vi "AttackedSquares.vi"(10 "Turn":T2, 11 "Input Squares":T1[][](array[typedef])) -> (3 "Attacked Squares":bool[][](array[boolean]))   [LabVIEW 2019]
doc: "This VI creates virtual chessboard with squares attacked by player that made last move"
uses:
  #typedef_Color.ctl
  #typedef_SquareType.ctl
  #typedef_Piece.ctl
  #typedef_PieceType.ctl
panel:
  out "?":u16[][](array[ring])
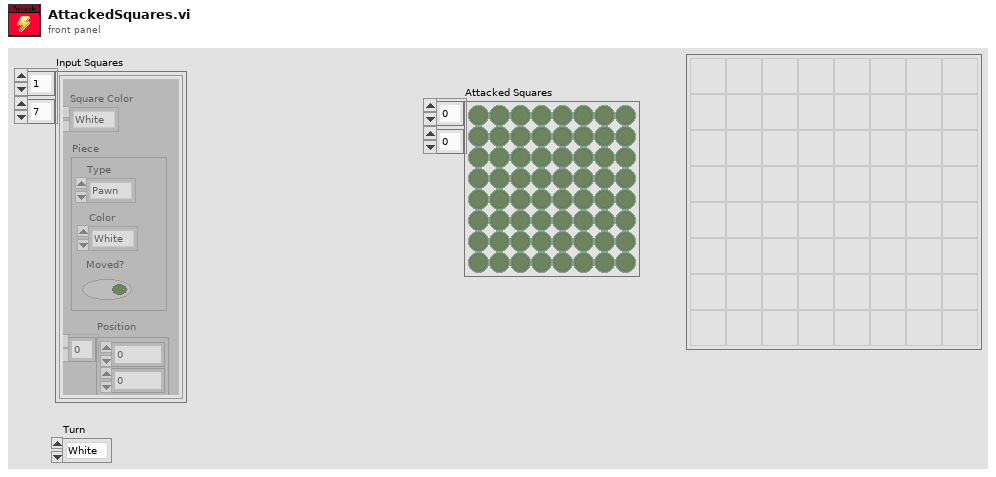
[diagram p1: front panel]
types:
  T1 = typedef "#typedef_SquareType.ctl" = cluster{"Square Color":T2, "Position":i32[], "Piece":T3}
  T2 = typedef "#typedef_Color.ctl" = enum16{"White", "Black"}
  T3 = typedef "#typedef_Piece.ctl" = cluster{"Type":T4, "Color":T2, "Moved?":bool}
  T4 = typedef "#typedef_PieceType.ctl" = enum16{"None", "Pawn", "Knight", "Bishop", "Rook", "Queen", "King"}
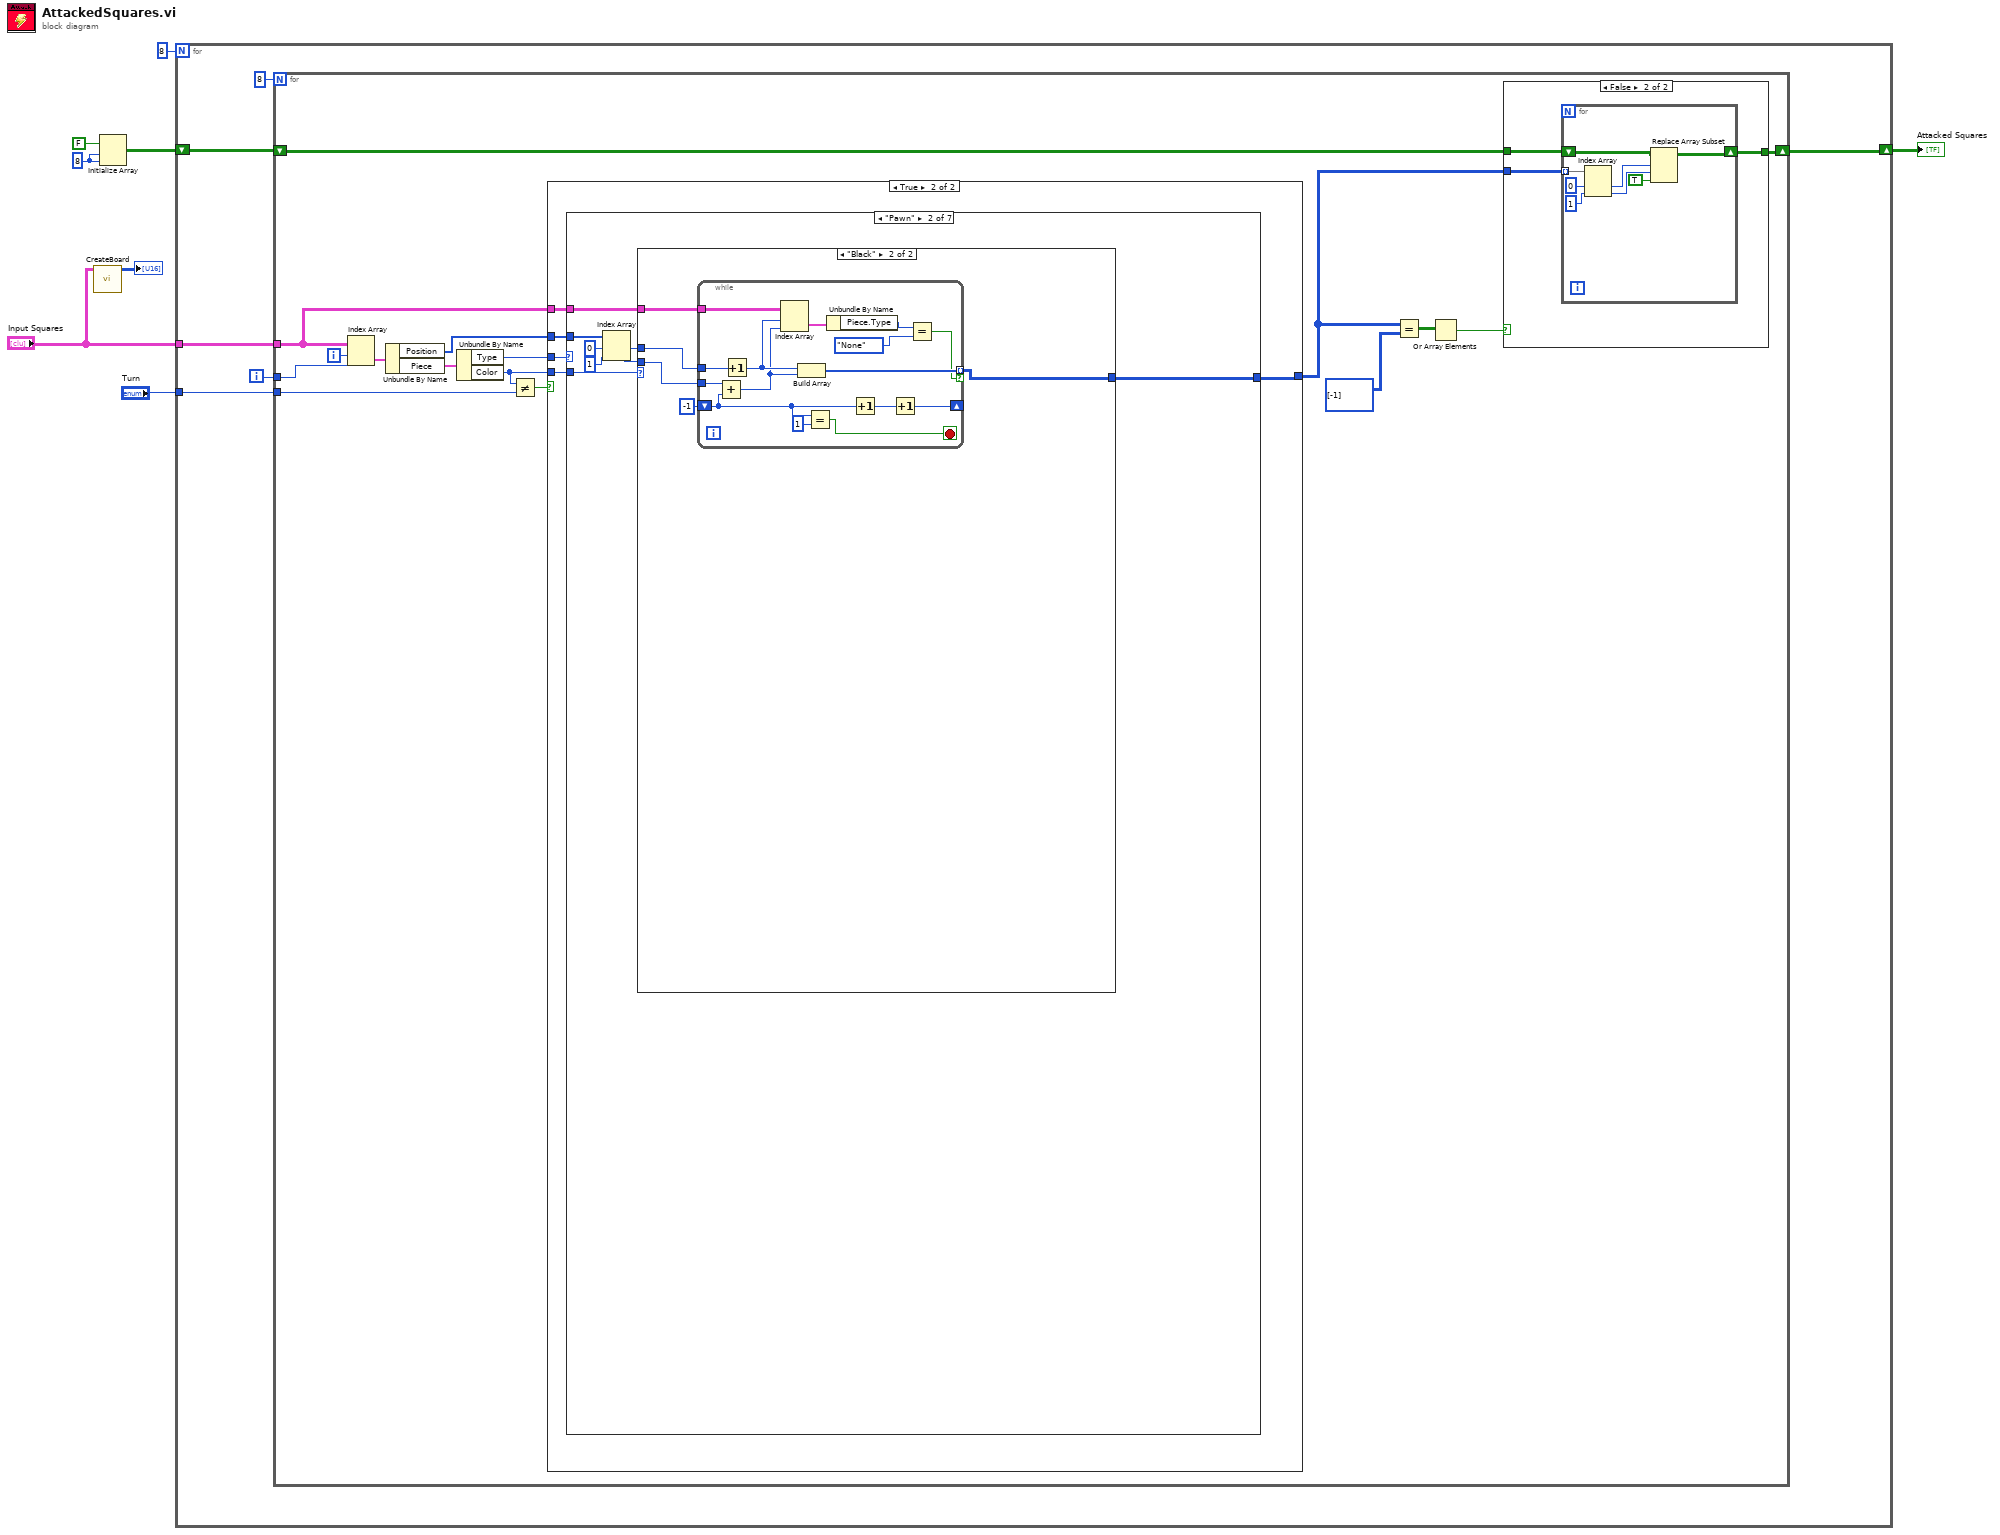
[diagram p0: block diagram]
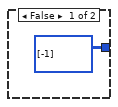
[diagram p3: hidden frame]
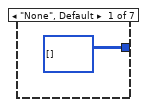
[diagram p4: hidden frame]
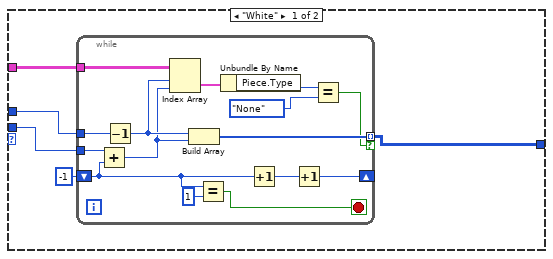
[diagram p5: hidden frame]
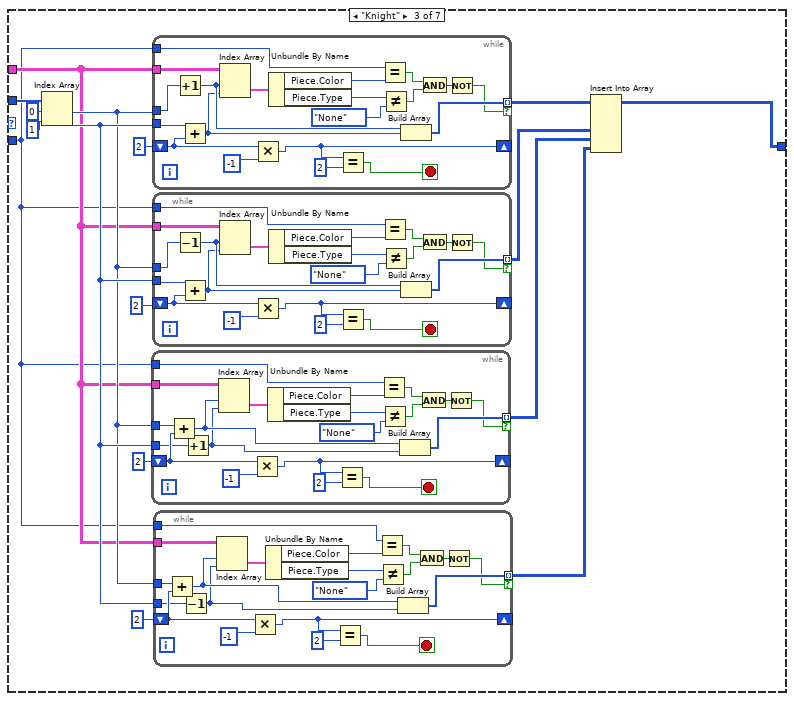
[diagram p6: hidden frame]
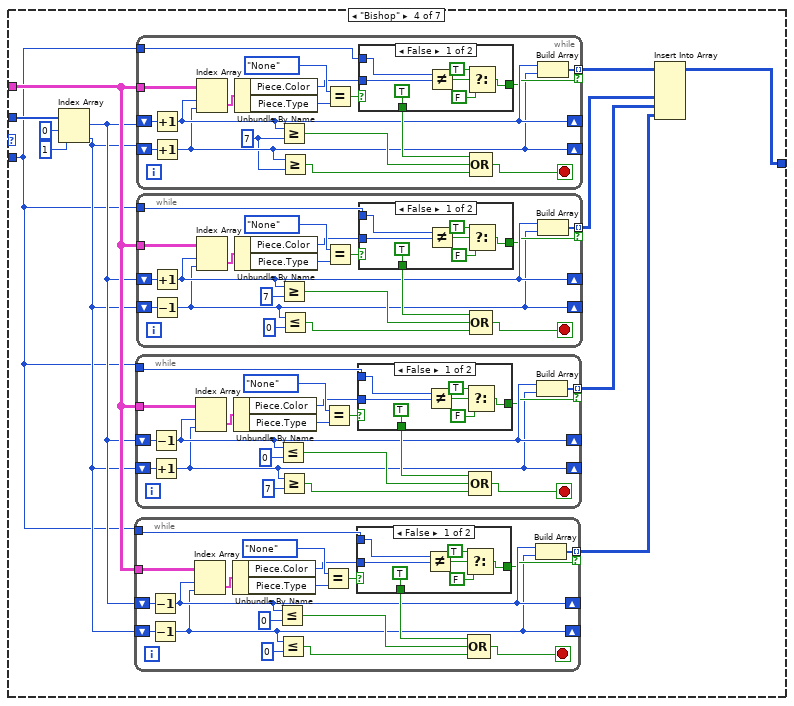
[diagram p7: hidden frame]
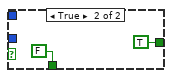
[diagram p8: hidden frame]
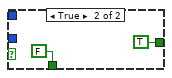
[diagram p9: hidden frame]
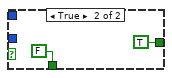
[diagram p10: hidden frame]
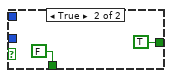
[diagram p11: hidden frame]
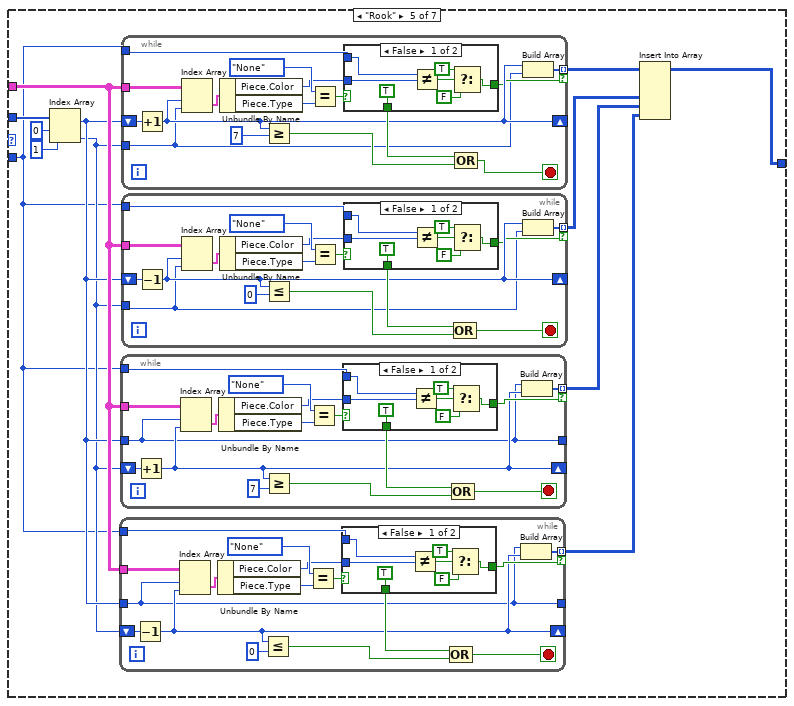
[diagram p12: hidden frame]
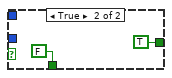
[diagram p13: hidden frame]
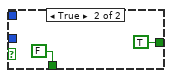
[diagram p14: hidden frame]
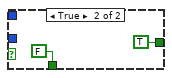
[diagram p15: hidden frame]
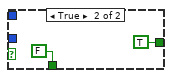
[diagram p16: hidden frame]
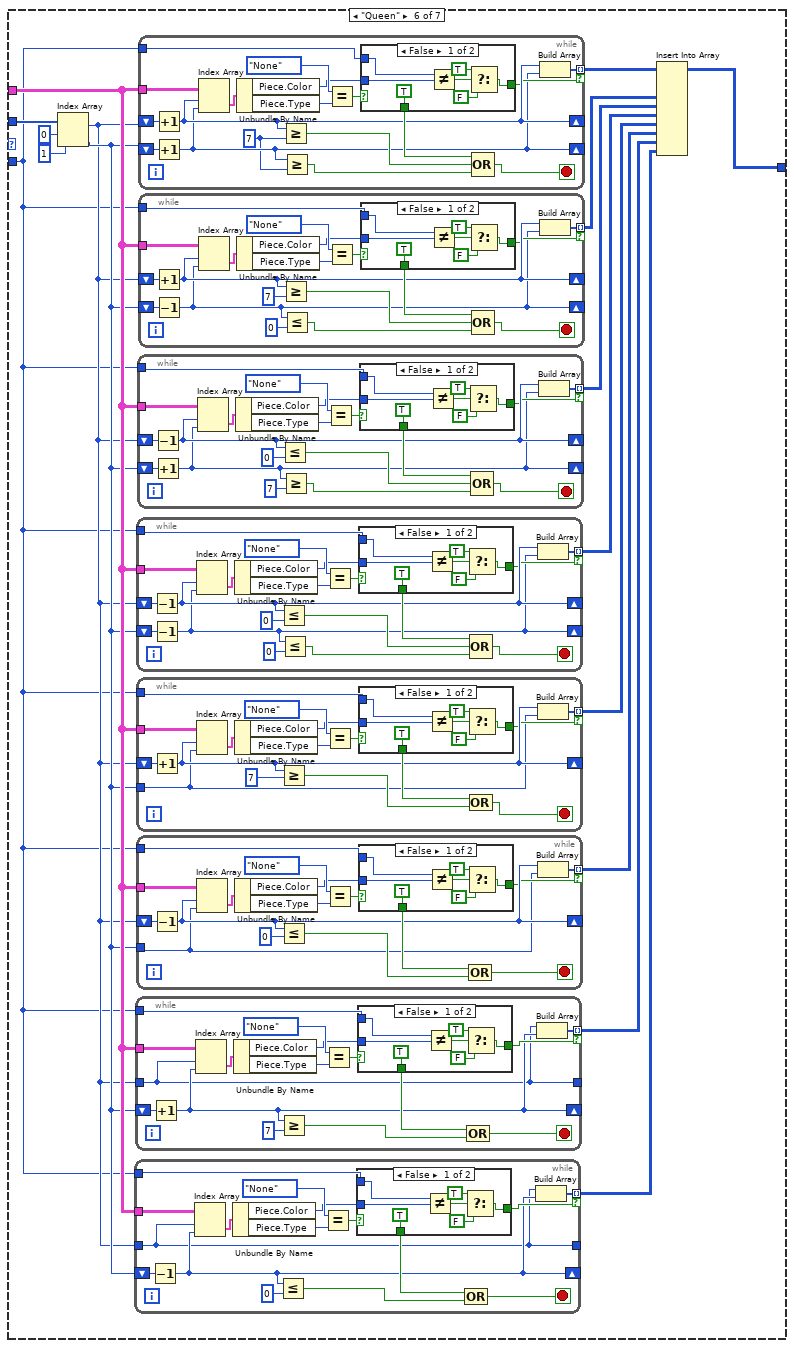
[diagram p17: hidden frame]
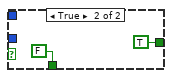
[diagram p18: hidden frame]
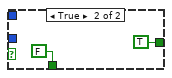
[diagram p19: hidden frame]
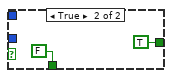
[diagram p20: hidden frame]
diagram:
  w5 = 8 ("dimension size")
  n1 = call "CreateBoard.vi"("Squares type"="Input Squares") -> ("Board"=→"?":u16[][])  [unwired: 10 in]
  n2 = Initialize Array(FALSE, w5, w5) -> (w6:bool[][])
  n3 = for {
    N: 8 -> [_]
    tunnel: "Input Squares" -> [w14]
    tunnel: "Turn" -> [w13]
    shift-right: [w10] -> w7
    shift-left: w6 -> [w11]
    i -> [w12]
    n4 = for {
      N: 8 -> [_]
      tunnel: w14 -> [w30]
      tunnel: w13 -> [w25]
      tunnel: w12 -> [w21]
      shift-right: [w15] -> w10
      shift-left: w11 -> [w17]
      i -> [w22]
      n5 = Index Array(array=w30, index (row)=w22, index (col)=w21) -> (element=w23:T1)
      n6 = Unbundle By Name(w23) -> ("Position"=w28:i32[], "Piece"=w24:T3)
      n7 = Unbundle By Name(w24) -> ("Type"=w27:T4, "Color"=w29:T2)
      n8 = Not Equal?(x=w29, y=w25) -> (x != y?=w26:bool)
      n9 = case shown="True" w26 {
        tunnel: w27 -> [_ w48]
        tunnel: w28 -> [_ w47]
        tunnel: w29 -> [_ w46]
        tunnel: w30 -> [_ w45]
        tunnel: [i32[][] [[-1]] w44] -> w16
        frame False {
        }
        frame True {
          n10 = case shown="\"Pawn\"" w48 {
            tunnel: w47 -> [_ w54 w100 w203 w326 w442 w669]
            tunnel: w46 -> [_ w57 w99 w195 w318 w434 w661]
            tunnel: w45 -> [_ w51 w101 w198 w321 w437 w664]
            tunnel: [i32[][] [] w50 w98 w194 w317 w429 w656] -> w44
            frame "None", Default {
            }
            frame "Pawn" {
              n11 = Index Array(array=w54, index #1=0 ("index"), index #2=1 ("index")) -> (element #1=w53:i32, element #2=w52:i32)
              n12 = case shown="\"Black\"" w57 {
                tunnel: w53 -> [w61 w81]
                tunnel: w52 -> [w60 w80]
                tunnel: w51 -> [w59 w79]
                tunnel: [w58 w78] -> w50
                frame "White" {
                  n13 = while {
                    tunnel: w61 -> [w73]
                    tunnel: w60 -> [w72]
                    tunnel: w59 -> [w70]
                    tunnel: [w64] -> w58 mode=indexing if=w63
                    shift-right: [w76] -> _
                    shift-left: -1 ("index") -> [w71]
                    stop <- w74 stop-if-true
                    n14 = Add(x=w72, y=w71) -> (x+y=w65:i32)
                    n15 = Decrement(x=w73) -> (x-1=w66:i32)
                    n16 = Index Array(array=w70, index (row)=w66, index (col)=w65) -> (element=w69:T1)
                    n17 = Build Array(w66, w65) -> (w64:i32[])
                    n18 = Equal?(x=w71, y=1) -> (x = y?=w74:bool)
                    n19 = Unbundle By Name(w69) -> ("Piece.Type"=w68:T4)
                    n20 = Increment(x=w71) -> (x+1=w77:i32)
                    n21 = Increment(x=w77) -> (x+1=w76:i32)
                    n22 = Equal?(x=w68, y=#typedef_PieceType."None") -> (x = y?=w63:bool)
                  }
                }
                frame "Black" {
                  n23 = while {
                    tunnel: w81 -> [w93]
                    tunnel: w80 -> [w92]
                    tunnel: w79 -> [w90]
                    tunnel: [w84] -> w78 mode=indexing if=w83
                    shift-right: [w96] -> _
                    shift-left: -1 ("index") -> [w91]
                    stop <- w94 stop-if-true
                    n24 = Add(x=w92, y=w91) -> (x+y=w85:i32)
                    n25 = Increment(x=w93) -> (x+1=w86:i32)
                    n26 = Index Array(array=w90, index (row)=w86, index (col)=w85) -> (element=w89:T1)
                    n27 = Build Array(w86, w85) -> (w84:i32[])
                    n28 = Equal?(x=w91, y=1) -> (x = y?=w94:bool)
                    n29 = Unbundle By Name(w89) -> ("Piece.Type"=w88:T4)
                    n30 = Increment(x=w91) -> (x+1=w97:i32)
                    n31 = Increment(x=w97) -> (x+1=w96:i32)
                    n32 = Equal?(x=w88, y=#typedef_PieceType."None") -> (x = y?=w83:bool)
                  }
                }
              }
            }
            frame "Knight" {
              n33 = Index Array(array=w100, index #1=0 ("index"), index #2=1 ("index")) -> (element #1=w106:i32, element #2=w107:i32)
              n34 = while {
                tunnel: w101 -> [w153]
                tunnel: w106 -> [w140]
                tunnel: w107 -> [w138]
                shift-right: [w146] -> _
                shift-left: 2 -> [w139]
                tunnel: [w143] -> w103 mode=indexing if=w141
                tunnel: w99 -> [w134]
                stop <- w144 stop-if-true
                n35 = Add(x=w140, y=w139) -> (x+y=w137:i32)
                n36 = Increment(x=w138) -> (x+1=w136:i32)
                n37 = Index Array(array=w153, index (row)=w137, index (col)=w136) -> (element=w151:T1)
                n38 = Multiply(x=w139, y=-1) -> (x*y=w146:i32)
                n39 = Unbundle By Name(w151) -> ("Piece.Color"=w150:T2, "Piece.Type"=w149:T4)
                n40 = Equal?(x=w146, y=2) -> (x = y?=w144:bool)
                n41 = Equal?(x=w134, y=w150) -> (x = y?=w148:bool)
                n42 = Not Equal?(x=w149, y=#typedef_PieceType."None") -> (x != y?=w147:bool)
                n43 = Build Array(w137, w136) -> (w143:i32[])
                n44 = And(x=w148, y=w147) -> (x .and. y?=w142:bool)
                n45 = Not(x=w142) -> (.not. x?=w141:bool)
              }
              n46 = while {
                tunnel: w101 -> [w193]
                tunnel: w106 -> [w189]
                tunnel: w107 -> [w190]
                shift-right: [w183] -> _
                shift-left: 2 -> [w191]
                tunnel: [w178] -> w105 mode=indexing if=w176
                tunnel: w99 -> [w174]
                stop <- w181 stop-if-true
                n47 = Increment(x=w189) -> (x+1=w180:i32)
                n48 = Add(x=w190, y=w191) -> (x+y=w179:i32)
                n49 = Index Array(array=w193, index (row)=w180, index (col)=w179) -> (element=w188:T1)
                n50 = Multiply(x=w191, y=-1) -> (x*y=w183:i32)
                n51 = Unbundle By Name(w188) -> ("Piece.Color"=w187:T2, "Piece.Type"=w186:T4)
                n52 = Equal?(x=w183, y=2) -> (x = y?=w181:bool)
                n53 = Equal?(x=w174, y=w187) -> (x = y?=w185:bool)
                n54 = Not Equal?(x=w186, y=#typedef_PieceType."None") -> (x != y?=w184:bool)
                n55 = Build Array(w180, w179) -> (w178:i32[])
                n56 = And(x=w185, y=w184) -> (x .and. y?=w177:bool)
                n57 = Not(x=w177) -> (.not. x?=w176:bool)
              }
              n58 = while {
                tunnel: w101 -> [w173]
                tunnel: w106 -> [w169]
                tunnel: w107 -> [w170]
                shift-right: [w163] -> _
                shift-left: 2 -> [w171]
                tunnel: [w158] -> w104 mode=indexing if=w156
                tunnel: w99 -> [w154]
                stop <- w161 stop-if-true
                n59 = Decrement(x=w169) -> (x-1=w160:i32)
                n60 = Add(x=w170, y=w171) -> (x+y=w159:i32)
                n61 = Index Array(array=w173, index (row)=w160, index (col)=w159) -> (element=w168:T1)
                n62 = Multiply(x=w171, y=-1) -> (x*y=w163:i32)
                n63 = Unbundle By Name(w168) -> ("Piece.Color"=w167:T2, "Piece.Type"=w166:T4)
                n64 = Equal?(x=w163, y=2) -> (x = y?=w161:bool)
                n65 = Equal?(x=w154, y=w167) -> (x = y?=w165:bool)
                n66 = Not Equal?(x=w166, y=#typedef_PieceType."None") -> (x != y?=w164:bool)
                n67 = Build Array(w160, w159) -> (w158:i32[])
                n68 = And(x=w165, y=w164) -> (x .and. y?=w157:bool)
                n69 = Not(x=w157) -> (.not. x?=w156:bool)
              }
              n70 = while {
                tunnel: w101 -> [w133]
                tunnel: w106 -> [w120]
                tunnel: w107 -> [w118]
                shift-right: [w126] -> _
                shift-left: 2 -> [w119]
                tunnel: [w123] -> w102 mode=indexing if=w121
                tunnel: w99 -> [w114]
                stop <- w124 stop-if-true
                n71 = Add(x=w120, y=w119) -> (x+y=w117:i32)
                n72 = Decrement(x=w118) -> (x-1=w116:i32)
                n73 = Index Array(array=w133, index (row)=w117, index (col)=w116) -> (element=w131:T1)
                n74 = Multiply(x=w119, y=-1) -> (x*y=w126:i32)
                n75 = Unbundle By Name(w131) -> ("Piece.Color"=w130:T2, "Piece.Type"=w129:T4)
                n76 = Equal?(x=w126, y=2) -> (x = y?=w124:bool)
                n77 = Equal?(x=w114, y=w130) -> (x = y?=w128:bool)
                n78 = Not Equal?(x=w129, y=#typedef_PieceType."None") -> (x != y?=w127:bool)
                n79 = Build Array(w117, w116) -> (w123:i32[])
                n80 = And(x=w128, y=w127) -> (x .and. y?=w122:bool)
                n81 = Not(x=w122) -> (.not. x?=w121:bool)
              }
              n82 = Insert Into Array(array=w105, new element #1=w104, new element #2=w103, new element #3=w102) -> (w98:i32[][])  [unwired: 2 in]
            }
            frame "Bishop" {
              n83 = Index Array(array=w203, index #1=0 ("index (row)"), index #2=1 ("index")) -> (element #1=w197:i32, element #2=w196:i32)
              n84 = while {
                tunnel: w198 -> [w222]
                shift-right: [w211] -> _
                shift-left: w197 -> [w223]
                shift-right: [w208] -> _
                shift-left: w196 -> [w224]
                tunnel: [w210] -> w199 mode=indexing if=w209
                tunnel: w195 -> [w206]
                stop <- w212 stop-if-true
                n85 = Decrement(x=w223) -> (x-1=w211:i32)
                n86 = Decrement(x=w224) -> (x-1=w208:i32)
                n87 = Index Array(array=w222, index (row)=w211, index (col)=w208) -> (element=w221:T1)
                n88 = Unbundle By Name(w221) -> ("Piece.Color"=w217:T2, "Piece.Type"=w220:T4)
                n89 = Less Or Equal?(x=w211, y=0) -> (x <= y?=w214:bool)
                n90 = Less Or Equal?(x=w208, y=0) -> (x <= y?=w213:bool)
                n91 = Equal?(x=#typedef_PieceType."None", y=w220) -> (x = y?=w218:bool)
                n92 = case shown="False" w218 {
                  tunnel: w217 -> [w231 _]
                  tunnel: [TRUE FALSE] -> w215
                  tunnel: [w226 TRUE] -> w209
                  tunnel: w206 -> [w225 _]
                  frame False {
                    n93 = Not Equal?(x=w225, y=w231) -> (x != y?=w229:bool)
                    n94 = Select(t=TRUE, s=w229, f=FALSE) -> (s? t:f=w226:bool)
                  }
                  frame True {
                  }
                }
                n95 = Compound Arithmetic op=OR(w215, w214, w213) -> (w212:bool)
                n96 = Build Array(w211, w208) -> (w210:i32[])
              }
              n97 = while {
                tunnel: w198 -> [w250]
                shift-right: [w239] -> _
                shift-left: w197 -> [w251]
                shift-right: [w236] -> _
                shift-left: w196 -> [w252]
                tunnel: [w238] -> w200 mode=indexing if=w237
                tunnel: w195 -> [w234]
                stop <- w240 stop-if-true
                n98 = Decrement(x=w251) -> (x-1=w239:i32)
                n99 = Increment(x=w252) -> (x+1=w236:i32)
                n100 = Index Array(array=w250, index (row)=w239, index (col)=w236) -> (element=w249:T1)
                n101 = Unbundle By Name(w249) -> ("Piece.Color"=w245:T2, "Piece.Type"=w248:T4)
                n102 = Less Or Equal?(x=w239, y=0) -> (x <= y?=w242:bool)
                n103 = Greater Or Equal?(x=w236, y=7) -> (x >= y?=w241:bool)
                n104 = Equal?(x=#typedef_PieceType."None", y=w248) -> (x = y?=w246:bool)
                n105 = case shown="False" w246 {
                  tunnel: w245 -> [w259 _]
                  tunnel: [TRUE FALSE] -> w243
                  tunnel: [w254 TRUE] -> w237
                  tunnel: w234 -> [w253 _]
                  frame False {
                    n106 = Not Equal?(x=w253, y=w259) -> (x != y?=w257:bool)
                    n107 = Select(t=TRUE, s=w257, f=FALSE) -> (s? t:f=w254:bool)
                  }
                  frame True {
                  }
                }
                n108 = Compound Arithmetic op=OR(w243, w242, w241) -> (w240:bool)
                n109 = Build Array(w239, w236) -> (w238:i32[])
              }
              n110 = while {
                tunnel: w198 -> [w305]
                shift-right: [w295] -> _
                shift-left: w197 -> [w306]
                shift-right: [w292] -> _
                shift-left: w196 -> [w307]
                tunnel: [w294] -> w202 mode=indexing if=w293
                tunnel: w195 -> [w290]
                stop <- w296 stop-if-true
                w291 = 7 ("y")
                n111 = Increment(x=w306) -> (x+1=w295:i32)
                n112 = Increment(x=w307) -> (x+1=w292:i32)
                n113 = Index Array(array=w305, index (row)=w295, index (col)=w292) -> (element=w304:T1)
                n114 = Unbundle By Name(w304) -> ("Piece.Color"=w300:T2, "Piece.Type"=w303:T4)
                n115 = Greater Or Equal?(x=w295, y=w291) -> (x >= y?=w298:bool)
                n116 = Greater Or Equal?(x=w292, y=w291) -> (x >= y?=w297:bool)
                n117 = Equal?(x=#typedef_PieceType."None", y=w303) -> (x = y?=w301:bool)
                n118 = case shown="False" w301 {
                  tunnel: w300 -> [w314 _]
                  tunnel: [TRUE FALSE] -> w299
                  tunnel: [w309 TRUE] -> w293
                  tunnel: w290 -> [w308 _]
                  frame False {
                    n119 = Not Equal?(x=w308, y=w314) -> (x != y?=w312:bool)
                    n120 = Select(t=TRUE, s=w312, f=FALSE) -> (s? t:f=w309:bool)
                  }
                  frame True {
                  }
                }
                n121 = Compound Arithmetic op=OR(w299, w298, w297) -> (w296:bool)
                n122 = Build Array(w295, w292) -> (w294:i32[])
              }
              n123 = while {
                tunnel: w198 -> [w278]
                shift-right: [w267] -> _
                shift-left: w197 -> [w279]
                shift-right: [w264] -> _
                shift-left: w196 -> [w280]
                tunnel: [w266] -> w201 mode=indexing if=w265
                tunnel: w195 -> [w262]
                stop <- w268 stop-if-true
                n124 = Increment(x=w279) -> (x+1=w267:i32)
                n125 = Decrement(x=w280) -> (x-1=w264:i32)
                n126 = Index Array(array=w278, index (row)=w267, index (col)=w264) -> (element=w277:T1)
                n127 = Unbundle By Name(w277) -> ("Piece.Color"=w273:T2, "Piece.Type"=w276:T4)
                n128 = Greater Or Equal?(x=w267, y=7) -> (x >= y?=w270:bool)
                n129 = Less Or Equal?(x=w264, y=0) -> (x <= y?=w269:bool)
                n130 = Equal?(x=#typedef_PieceType."None", y=w276) -> (x = y?=w274:bool)
                n131 = case shown="False" w274 {
                  tunnel: w273 -> [w287 _]
                  tunnel: [TRUE FALSE] -> w271
                  tunnel: [w282 TRUE] -> w265
                  tunnel: w262 -> [w281 _]
                  frame False {
                    n132 = Not Equal?(x=w281, y=w287) -> (x != y?=w285:bool)
                    n133 = Select(t=TRUE, s=w285, f=FALSE) -> (s? t:f=w282:bool)
                  }
                  frame True {
                  }
                }
                n134 = Compound Arithmetic op=OR(w271, w270, w269) -> (w268:bool)
                n135 = Build Array(w267, w264) -> (w266:i32[])
              }
              n136 = Insert Into Array(array=w202, new element #1=w201, new element #2=w200, new element #3=w199) -> (w194:i32[][])  [unwired: 2 in]
            }
            frame "Rook" {
              n137 = Index Array(array=w326, index #1=0 ("index (row)"), index #2=1 ("index")) -> (element #1=w320:i32, element #2=w319:i32)
              n138 = while {
                tunnel: w321 -> [w343]
                shift-right: [w333] -> _
                shift-left: w319 -> [w344]
                tunnel: [w335] -> w322 mode=indexing if=w334
                tunnel: w320 -> [w331]
                tunnel: [w331] -> _
                tunnel: w318 -> [w329]
                stop <- w336 stop-if-true
                n139 = Decrement(x=w344) -> (x-1=w333:i32)
                n140 = Index Array(array=w343, index (row)=w331, index (col)=w333) -> (element=w342:T1)
                n141 = Unbundle By Name(w342) -> ("Piece.Color"=w338:T2, "Piece.Type"=w341:T4)
                n142 = Less Or Equal?(x=w333, y=0) -> (x <= y?=w330:bool)
                n143 = Equal?(x=#typedef_PieceType."None", y=w341) -> (x = y?=w339:bool)
                n144 = case shown="False" w339 {
                  tunnel: w338 -> [w351 _]
                  tunnel: [TRUE FALSE] -> w337
                  tunnel: [w346 TRUE] -> w334
                  tunnel: w329 -> [w345 _]
                  frame False {
                    n145 = Not Equal?(x=w345, y=w351) -> (x != y?=w349:bool)
                    n146 = Select(t=TRUE, s=w349, f=FALSE) -> (s? t:f=w346:bool)
                  }
                  frame True {
                  }
                }
                n147 = Compound Arithmetic op=OR(w337, w330) -> (w336:bool)
                n148 = Build Array(w331, w333) -> (w335:i32[])
              }
              n149 = while {
                tunnel: w321 -> [w368]
                shift-right: [w358] -> _
                shift-left: w319 -> [w369]
                tunnel: [w360] -> w323 mode=indexing if=w359
                tunnel: w320 -> [w356]
                tunnel: [w356] -> _
                tunnel: w318 -> [w354]
                stop <- w361 stop-if-true
                n150 = Increment(x=w369) -> (x+1=w358:i32)
                n151 = Index Array(array=w368, index (row)=w356, index (col)=w358) -> (element=w367:T1)
                n152 = Unbundle By Name(w367) -> ("Piece.Color"=w363:T2, "Piece.Type"=w366:T4)
                n153 = Greater Or Equal?(x=w358, y=7) -> (x >= y?=w355:bool)
                n154 = Equal?(x=#typedef_PieceType."None", y=w366) -> (x = y?=w364:bool)
                n155 = case shown="False" w364 {
                  tunnel: w363 -> [w376 _]
                  tunnel: [TRUE FALSE] -> w362
                  tunnel: [w371 TRUE] -> w359
                  tunnel: w354 -> [w370 _]
                  frame False {
                    n156 = Not Equal?(x=w370, y=w376) -> (x != y?=w374:bool)
                    n157 = Select(t=TRUE, s=w374, f=FALSE) -> (s? t:f=w371:bool)
                  }
                  frame True {
                  }
                }
                n158 = Compound Arithmetic op=OR(w362, w355) -> (w361:bool)
                n159 = Build Array(w356, w358) -> (w360:i32[])
              }
              n160 = while {
                tunnel: w321 -> [w418]
                shift-right: [w409] -> _
                shift-left: w320 -> [w419]
                tunnel: [w408] -> w325 mode=indexing if=w407
                tunnel: w319 -> [w405]
                tunnel: w318 -> [w404]
                stop <- w410 stop-if-true
                n161 = Increment(x=w419) -> (x+1=w409:i32)
                n162 = Index Array(array=w418, index (row)=w409, index (col)=w405) -> (element=w417:T1)
                n163 = Unbundle By Name(w417) -> ("Piece.Color"=w413:T2, "Piece.Type"=w416:T4)
                n164 = Greater Or Equal?(x=w409, y=7) -> (x >= y?=w411:bool)
                n165 = Equal?(x=#typedef_PieceType."None", y=w416) -> (x = y?=w414:bool)
                n166 = case shown="False" w414 {
                  tunnel: w413 -> [w426 _]
                  tunnel: [TRUE FALSE] -> w412
                  tunnel: [w421 TRUE] -> w407
                  tunnel: w404 -> [w420 _]
                  frame False {
                    n167 = Not Equal?(x=w420, y=w426) -> (x != y?=w424:bool)
                    n168 = Select(t=TRUE, s=w424, f=FALSE) -> (s? t:f=w421:bool)
                  }
                  frame True {
                  }
                }
                n169 = Compound Arithmetic op=OR(w412, w411) -> (w410:bool)
                n170 = Build Array(w409, w405) -> (w408:i32[])
              }
              n171 = while {
                tunnel: w321 -> [w393]
                shift-right: [w383] -> _
                shift-left: w320 -> [w394]
                tunnel: [w382] -> w324 mode=indexing if=w381
                tunnel: w319 -> [w380]
                tunnel: w318 -> [w379]
                stop <- w384 stop-if-true
                n172 = Decrement(x=w394) -> (x-1=w383:i32)
                n173 = Index Array(array=w393, index (row)=w383, index (col)=w380) -> (element=w392:T1)
                n174 = Unbundle By Name(w392) -> ("Piece.Color"=w388:T2, "Piece.Type"=w391:T4)
                n175 = Less Or Equal?(x=w383, y=0) -> (x <= y?=w385:bool)
                n176 = Equal?(x=#typedef_PieceType."None", y=w391) -> (x = y?=w389:bool)
                n177 = case shown="False" w389 {
                  tunnel: w388 -> [w401 _]
                  tunnel: [TRUE FALSE] -> w386
                  tunnel: [w396 TRUE] -> w381
                  tunnel: w379 -> [w395 _]
                  frame False {
                    n178 = Not Equal?(x=w395, y=w401) -> (x != y?=w399:bool)
                    n179 = Select(t=TRUE, s=w399, f=FALSE) -> (s? t:f=w396:bool)
                  }
                  frame True {
                  }
                }
                n180 = Compound Arithmetic op=OR(w386, w385) -> (w384:bool)
                n181 = Build Array(w383, w380) -> (w382:i32[])
              }
              n182 = Insert Into Array(array=w325, new element #1=w324, new element #2=w323, new element #3=w322) -> (w317:i32[][])  [unwired: 2 in]
            }
            frame "Queen" {
              n183 = Index Array(array=w442, index #1=0 ("index (row)"), index #2=1 ("index")) -> (element #1=w435:i32, element #2=w436:i32)
              n184 = while {
                tunnel: w437 -> [w459]
                shift-right: [w449] -> _
                shift-left: w436 -> [w460]
                tunnel: [w451] -> w430 mode=indexing if=w450
                tunnel: w435 -> [w447]
                tunnel: [w447] -> _
                tunnel: w434 -> [w445]
                stop <- w452 stop-if-true
                n185 = Decrement(x=w460) -> (x-1=w449:i32)
                n186 = Index Array(array=w459, index (row)=w447, index (col)=w449) -> (element=w458:T1)
                n187 = Unbundle By Name(w458) -> ("Piece.Color"=w454:T2, "Piece.Type"=w457:T4)
                n188 = Less Or Equal?(x=w449, y=0) -> (x <= y?=w446:bool)
                n189 = Equal?(x=#typedef_PieceType."None", y=w457) -> (x = y?=w455:bool)
                n190 = case shown="False" w455 {
                  tunnel: w454 -> [w467 _]
                  tunnel: [TRUE FALSE] -> w453
                  tunnel: [w462 TRUE] -> w450
                  tunnel: w445 -> [w461 _]
                  frame False {
                    n191 = Not Equal?(x=w461, y=w467) -> (x != y?=w465:bool)
                    n192 = Select(t=TRUE, s=w465, f=FALSE) -> (s? t:f=w462:bool)
                  }
                  frame True {
                  }
                }
                n193 = Compound Arithmetic op=OR(w453, w446) -> (w452:bool)
                n194 = Build Array(w447, w449) -> (w451:i32[])
              }
              n195 = while {
                tunnel: w437 -> [w484]
                shift-right: [w474] -> _
                shift-left: w436 -> [w485]
                tunnel: [w476] -> w431 mode=indexing if=w475
                tunnel: w435 -> [w472]
                tunnel: [w472] -> _
                tunnel: w434 -> [w470]
                stop <- w477 stop-if-true
                n196 = Increment(x=w485) -> (x+1=w474:i32)
                n197 = Index Array(array=w484, index (row)=w472, index (col)=w474) -> (element=w483:T1)
                n198 = Unbundle By Name(w483) -> ("Piece.Color"=w479:T2, "Piece.Type"=w482:T4)
                n199 = Greater Or Equal?(x=w474, y=7) -> (x >= y?=w471:bool)
                n200 = Equal?(x=#typedef_PieceType."None", y=w482) -> (x = y?=w480:bool)
                n201 = case shown="False" w480 {
                  tunnel: w479 -> [w492 _]
                  tunnel: [TRUE FALSE] -> w478
                  tunnel: [w487 TRUE] -> w475
                  tunnel: w470 -> [w486 _]
                  frame False {
                    n202 = Not Equal?(x=w486, y=w492) -> (x != y?=w490:bool)
                    n203 = Select(t=TRUE, s=w490, f=FALSE) -> (s? t:f=w487:bool)
                  }
                  frame True {
                  }
                }
                n204 = Compound Arithmetic op=OR(w478, w471) -> (w477:bool)
                n205 = Build Array(w472, w474) -> (w476:i32[])
              }
              n206 = while {
                tunnel: w437 -> [w561]
                shift-right: [w550] -> _
                shift-left: w435 -> [w562]
                shift-right: [w547] -> _
                shift-left: w436 -> [w563]
                tunnel: [w549] -> w438 mode=indexing if=w548
                tunnel: w434 -> [w545]
                stop <- w551 stop-if-true
                n207 = Decrement(x=w562) -> (x-1=w550:i32)
                n208 = Decrement(x=w563) -> (x-1=w547:i32)
                n209 = Index Array(array=w561, index (row)=w550, index (col)=w547) -> (element=w560:T1)
                n210 = Unbundle By Name(w560) -> ("Piece.Color"=w556:T2, "Piece.Type"=w559:T4)
                n211 = Less Or Equal?(x=w550, y=0) -> (x <= y?=w553:bool)
                n212 = Less Or Equal?(x=w547, y=0) -> (x <= y?=w552:bool)
                n213 = Equal?(x=#typedef_PieceType."None", y=w559) -> (x = y?=w557:bool)
                n214 = case shown="False" w557 {
                  tunnel: w556 -> [w570 _]
                  tunnel: [TRUE FALSE] -> w554
                  tunnel: [w565 TRUE] -> w548
                  tunnel: w545 -> [w564 _]
                  frame False {
                    n215 = Not Equal?(x=w564, y=w570) -> (x != y?=w568:bool)
                    n216 = Select(t=TRUE, s=w568, f=FALSE) -> (s? t:f=w565:bool)
                  }
                  frame True {
                  }
                }
                n217 = Compound Arithmetic op=OR(w554, w553, w552) -> (w551:bool)
                n218 = Build Array(w550, w547) -> (w549:i32[])
              }
              n219 = while {
                tunnel: w437 -> [w534]
                shift-right: [w525] -> _
                shift-left: w435 -> [w535]
                tunnel: [w524] -> w433 mode=indexing if=w523
                tunnel: w436 -> [w521]
                tunnel: w434 -> [w520]
                stop <- w526 stop-if-true
                n220 = Increment(x=w535) -> (x+1=w525:i32)
                n221 = Index Array(array=w534, index (row)=w525, index (col)=w521) -> (element=w533:T1)
                n222 = Unbundle By Name(w533) -> ("Piece.Color"=w529:T2, "Piece.Type"=w532:T4)
                n223 = Greater Or Equal?(x=w525, y=7) -> (x >= y?=w527:bool)
                n224 = Equal?(x=#typedef_PieceType."None", y=w532) -> (x = y?=w530:bool)
                n225 = case shown="False" w530 {
                  tunnel: w529 -> [w542 _]
                  tunnel: [TRUE FALSE] -> w528
                  tunnel: [w537 TRUE] -> w523
                  tunnel: w520 -> [w536 _]
                  frame False {
                    n226 = Not Equal?(x=w536, y=w542) -> (x != y?=w540:bool)
                    n227 = Select(t=TRUE, s=w540, f=FALSE) -> (s? t:f=w537:bool)
                  }
                  frame True {
                  }
                }
                n228 = Compound Arithmetic op=OR(w528, w527) -> (w526:bool)
                n229 = Build Array(w525, w521) -> (w524:i32[])
              }
              n230 = while {
                tunnel: w437 -> [w509]
                shift-right: [w499] -> _
                shift-left: w435 -> [w510]
                tunnel: [w498] -> w432 mode=indexing if=w497
                tunnel: w436 -> [w496]
                tunnel: w434 -> [w495]
                stop <- w500 stop-if-true
                n231 = Decrement(x=w510) -> (x-1=w499:i32)
                n232 = Index Array(array=w509, index (row)=w499, index (col)=w496) -> (element=w508:T1)
                n233 = Unbundle By Name(w508) -> ("Piece.Color"=w504:T2, "Piece.Type"=w507:T4)
                n234 = Less Or Equal?(x=w499, y=0) -> (x <= y?=w501:bool)
                n235 = Equal?(x=#typedef_PieceType."None", y=w507) -> (x = y?=w505:bool)
                n236 = case shown="False" w505 {
                  tunnel: w504 -> [w517 _]
                  tunnel: [TRUE FALSE] -> w502
                  tunnel: [w512 TRUE] -> w497
                  tunnel: w495 -> [w511 _]
                  frame False {
                    n237 = Not Equal?(x=w511, y=w517) -> (x != y?=w515:bool)
                    n238 = Select(t=TRUE, s=w515, f=FALSE) -> (s? t:f=w512:bool)
                  }
                  frame True {
                  }
                }
                n239 = Compound Arithmetic op=OR(w502, w501) -> (w500:bool)
                n240 = Build Array(w499, w496) -> (w498:i32[])
              }
              n241 = while {
                tunnel: w437 -> [w589]
                shift-right: [w578] -> _
                shift-left: w435 -> [w590]
                shift-right: [w575] -> _
                shift-left: w436 -> [w591]
                tunnel: [w577] -> w439 mode=indexing if=w576
                tunnel: w434 -> [w573]
                stop <- w579 stop-if-true
                n242 = Decrement(x=w590) -> (x-1=w578:i32)
                n243 = Increment(x=w591) -> (x+1=w575:i32)
                n244 = Index Array(array=w589, index (row)=w578, index (col)=w575) -> (element=w588:T1)
                n245 = Unbundle By Name(w588) -> ("Piece.Color"=w584:T2, "Piece.Type"=w587:T4)
                n246 = Less Or Equal?(x=w578, y=0) -> (x <= y?=w581:bool)
                n247 = Greater Or Equal?(x=w575, y=7) -> (x >= y?=w580:bool)
                n248 = Equal?(x=#typedef_PieceType."None", y=w587) -> (x = y?=w585:bool)
                n249 = case shown="False" w585 {
                  tunnel: w584 -> [w598 _]
                  tunnel: [TRUE FALSE] -> w582
                  tunnel: [w593 TRUE] -> w576
                  tunnel: w573 -> [w592 _]
                  frame False {
                    n250 = Not Equal?(x=w592, y=w598) -> (x != y?=w596:bool)
                    n251 = Select(t=TRUE, s=w596, f=FALSE) -> (s? t:f=w593:bool)
                  }
                  frame True {
                  }
                }
                n252 = Compound Arithmetic op=OR(w582, w581, w580) -> (w579:bool)
                n253 = Build Array(w578, w575) -> (w577:i32[])
              }
              n254 = while {
                tunnel: w437 -> [w644]
                shift-right: [w634] -> _
                shift-left: w435 -> [w645]
                shift-right: [w631] -> _
                shift-left: w436 -> [w646]
                tunnel: [w633] -> w441 mode=indexing if=w632
                tunnel: w434 -> [w629]
                stop <- w635 stop-if-true
                w630 = 7 ("y")
                n255 = Increment(x=w645) -> (x+1=w634:i32)
                n256 = Increment(x=w646) -> (x+1=w631:i32)
                n257 = Index Array(array=w644, index (row)=w634, index (col)=w631) -> (element=w643:T1)
                n258 = Unbundle By Name(w643) -> ("Piece.Color"=w639:T2, "Piece.Type"=w642:T4)
                n259 = Greater Or Equal?(x=w634, y=w630) -> (x >= y?=w637:bool)
                n260 = Greater Or Equal?(x=w631, y=w630) -> (x >= y?=w636:bool)
                n261 = Equal?(x=#typedef_PieceType."None", y=w642) -> (x = y?=w640:bool)
                n262 = case shown="False" w640 {
                  tunnel: w639 -> [w653 _]
                  tunnel: [TRUE FALSE] -> w638
                  tunnel: [w648 TRUE] -> w632
                  tunnel: w629 -> [w647 _]
                  frame False {
                    n263 = Not Equal?(x=w647, y=w653) -> (x != y?=w651:bool)
                    n264 = Select(t=TRUE, s=w651, f=FALSE) -> (s? t:f=w648:bool)
                  }
                  frame True {
                  }
                }
                n265 = Compound Arithmetic op=OR(w638, w637, w636) -> (w635:bool)
                n266 = Build Array(w634, w631) -> (w633:i32[])
              }
              n267 = while {
                tunnel: w437 -> [w617]
                shift-right: [w606] -> _
                shift-left: w435 -> [w618]
                shift-right: [w603] -> _
                shift-left: w436 -> [w619]
                tunnel: [w605] -> w440 mode=indexing if=w604
                tunnel: w434 -> [w601]
                stop <- w607 stop-if-true
                n268 = Increment(x=w618) -> (x+1=w606:i32)
                n269 = Decrement(x=w619) -> (x-1=w603:i32)
                n270 = Index Array(array=w617, index (row)=w606, index (col)=w603) -> (element=w616:T1)
                n271 = Unbundle By Name(w616) -> ("Piece.Color"=w612:T2, "Piece.Type"=w615:T4)
                n272 = Greater Or Equal?(x=w606, y=7) -> (x >= y?=w609:bool)
                n273 = Less Or Equal?(x=w603, y=0) -> (x <= y?=w608:bool)
                n274 = Equal?(x=#typedef_PieceType."None", y=w615) -> (x = y?=w613:bool)
                n275 = case shown="False" w613 {
                  tunnel: w612 -> [w626 _]
                  tunnel: [TRUE FALSE] -> w610
                  tunnel: [w621 TRUE] -> w604
                  tunnel: w601 -> [w620 _]
                  frame False {
                    n276 = Not Equal?(x=w620, y=w626) -> (x != y?=w624:bool)
                    n277 = Select(t=TRUE, s=w624, f=FALSE) -> (s? t:f=w621:bool)
                  }
                  frame True {
                  }
                }
                n278 = Compound Arithmetic op=OR(w610, w609, w608) -> (w607:bool)
                n279 = Build Array(w606, w603) -> (w605:i32[])
              }
              n280 = Insert Into Array(array=w441, new element #1=w440, new element #2=w439, new element #3=w438, new element #4=w433, new element #5=w432, new element #6=w431, new element #7=w430) -> (w429:i32[][])  [unwired: 2 in]
            }
            frame "King" {
              n281 = Index Array(array=w669, index #1=0 ("index (row)"), index #2=1 ("index")) -> (element #1=w662:i32, element #2=w663:i32)
              n282 = while {
                tunnel: w664 -> [w685]
                shift-right: [w675] -> _
                shift-left: w663 -> [w686]
                tunnel: [w677] -> w657 mode=indexing if=w676
                tunnel: w662 -> [w674]
                tunnel: [w674] -> _
                tunnel: w661 -> [w673]
                stop <- w678 stop-if-true
                n283 = Decrement(x=w686) -> (x-1=w675:i32)
                n284 = Index Array(array=w685, index (row)=w674, index (col)=w675) -> (element=w684:T1)
                n285 = Unbundle By Name(w684) -> ("Piece.Color"=w680:T2, "Piece.Type"=w683:T4)
                n286 = Equal?(x=#typedef_PieceType."None", y=w683) -> (x = y?=w681:bool)
                n287 = case shown="False" w681 {
                  tunnel: w680 -> [w693 _]
                  tunnel: [TRUE FALSE] -> w679
                  tunnel: [w688 TRUE] -> w676
                  tunnel: w673 -> [w687 _]
                  frame False {
                    n288 = Not Equal?(x=w687, y=w693) -> (x != y?=w691:bool)
                    n289 = Select(t=TRUE, s=w691, f=FALSE) -> (s? t:f=w688:bool)
                  }
                  frame True {
                  }
                }
                n290 = Compound Arithmetic op=OR(w679, TRUE ("value")) -> (w678:bool)
                n291 = Build Array(w674, w675) -> (w677:i32[])
              }
              n292 = while {
                tunnel: w664 -> [w709]
                shift-right: [w699] -> _
                shift-left: w663 -> [w710]
                tunnel: [w701] -> w658 mode=indexing if=w700
                tunnel: w662 -> [w698]
                tunnel: [w698] -> _
                tunnel: w661 -> [w697]
                stop <- w702 stop-if-true
                n293 = Increment(x=w710) -> (x+1=w699:i32)
                n294 = Index Array(array=w709, index (row)=w698, index (col)=w699) -> (element=w708:T1)
                n295 = Unbundle By Name(w708) -> ("Piece.Color"=w704:T2, "Piece.Type"=w707:T4)
                n296 = Equal?(x=#typedef_PieceType."None", y=w707) -> (x = y?=w705:bool)
                n297 = case shown="False" w705 {
                  tunnel: w704 -> [w717 _]
                  tunnel: [TRUE FALSE] -> w703
                  tunnel: [w712 TRUE] -> w700
                  tunnel: w697 -> [w711 _]
                  frame False {
                    n298 = Not Equal?(x=w711, y=w717) -> (x != y?=w715:bool)
                    n299 = Select(t=TRUE, s=w715, f=FALSE) -> (s? t:f=w712:bool)
                  }
                  frame True {
                  }
                }
                n300 = Compound Arithmetic op=OR(w703, TRUE ("value")) -> (w702:bool)
                n301 = Build Array(w698, w699) -> (w701:i32[])
              }
              n302 = while {
                tunnel: w664 -> [w781]
                shift-right: [w773] -> _
                shift-left: w662 -> [w782]
                shift-right: [w770] -> _
                shift-left: w663 -> [w783]
                tunnel: [w772] -> w665 mode=indexing if=w771
                tunnel: w661 -> [w769]
                stop <- w774 stop-if-true
                n303 = Decrement(x=w782) -> (x-1=w773:i32)
                n304 = Decrement(x=w783) -> (x-1=w770:i32)
                n305 = Index Array(array=w781, index (row)=w773, index (col)=w770) -> (element=w780:T1)
                n306 = Unbundle By Name(w780) -> ("Piece.Color"=w776:T2, "Piece.Type"=w779:T4)
                n307 = Equal?(x=#typedef_PieceType."None", y=w779) -> (x = y?=w777:bool)
                n308 = case shown="False" w777 {
                  tunnel: w776 -> [w790 _]
                  tunnel: [TRUE FALSE] -> w775
                  tunnel: [w785 TRUE] -> w771
                  tunnel: w769 -> [w784 _]
                  frame False {
                    n309 = Not Equal?(x=w784, y=w790) -> (x != y?=w788:bool)
                    n310 = Select(t=TRUE, s=w788, f=FALSE) -> (s? t:f=w785:bool)
                  }
                  frame True {
                  }
                }
                n311 = Compound Arithmetic op=OR(w775, TRUE ("value")) -> (w774:bool)
                n312 = Build Array(w773, w770) -> (w772:i32[])
              }
              n313 = while {
                tunnel: w664 -> [w757]
                shift-right: [w749] -> _
                shift-left: w662 -> [w758]
                tunnel: [w748] -> w660 mode=indexing if=w747
                tunnel: w663 -> [w746]
                tunnel: w661 -> [w745]
                stop <- w750 stop-if-true
                n314 = Increment(x=w758) -> (x+1=w749:i32)
                n315 = Index Array(array=w757, index (row)=w749, index (col)=w746) -> (element=w756:T1)
                n316 = Unbundle By Name(w756) -> ("Piece.Color"=w752:T2, "Piece.Type"=w755:T4)
                n317 = Equal?(x=#typedef_PieceType."None", y=w755) -> (x = y?=w753:bool)
                n318 = case shown="False" w753 {
                  tunnel: w752 -> [w765 _]
                  tunnel: [TRUE FALSE] -> w751
                  tunnel: [w760 TRUE] -> w747
                  tunnel: w745 -> [w759 _]
                  frame False {
                    n319 = Not Equal?(x=w759, y=w765) -> (x != y?=w763:bool)
                    n320 = Select(t=TRUE, s=w763, f=FALSE) -> (s? t:f=w760:bool)
                  }
                  frame True {
                  }
                }
                n321 = Compound Arithmetic op=OR(w751, TRUE ("value")) -> (w750:bool)
                n322 = Build Array(w749, w746) -> (w748:i32[])
              }
              n323 = while {
                tunnel: w664 -> [w733]
                shift-right: [w725] -> _
                shift-left: w662 -> [w734]
                tunnel: [w724] -> w659 mode=indexing if=w723
                tunnel: w663 -> [w722]
                tunnel: w661 -> [w721]
                stop <- w726 stop-if-true
                n324 = Decrement(x=w734) -> (x-1=w725:i32)
                n325 = Index Array(array=w733, index (row)=w725, index (col)=w722) -> (element=w732:T1)
                n326 = Unbundle By Name(w732) -> ("Piece.Color"=w728:T2, "Piece.Type"=w731:T4)
                n327 = Equal?(x=#typedef_PieceType."None", y=w731) -> (x = y?=w729:bool)
                n328 = case shown="False" w729 {
                  tunnel: w728 -> [w741 _]
                  tunnel: [TRUE FALSE] -> w727
                  tunnel: [w736 TRUE] -> w723
                  tunnel: w721 -> [w735 _]
                  frame False {
                    n329 = Not Equal?(x=w735, y=w741) -> (x != y?=w739:bool)
                    n330 = Select(t=TRUE, s=w739, f=FALSE) -> (s? t:f=w736:bool)
                  }
                  frame True {
                  }
                }
                n331 = Compound Arithmetic op=OR(w727, TRUE ("value")) -> (w726:bool)
                n332 = Build Array(w725, w722) -> (w724:i32[])
              }
              n333 = while {
                tunnel: w664 -> [w806]
                shift-right: [w798] -> _
                shift-left: w662 -> [w807]
                shift-right: [w795] -> _
                shift-left: w663 -> [w808]
                tunnel: [w797] -> w666 mode=indexing if=w796
                tunnel: w661 -> [w794]
                stop <- w799 stop-if-true
                n334 = Decrement(x=w807) -> (x-1=w798:i32)
                n335 = Increment(x=w808) -> (x+1=w795:i32)
                n336 = Index Array(array=w806, index (row)=w798, index (col)=w795) -> (element=w805:T1)
                n337 = Unbundle By Name(w805) -> ("Piece.Color"=w801:T2, "Piece.Type"=w804:T4)
                n338 = Equal?(x=#typedef_PieceType."None", y=w804) -> (x = y?=w802:bool)
                n339 = case shown="False" w802 {
                  tunnel: w801 -> [w815 _]
                  tunnel: [TRUE FALSE] -> w800
                  tunnel: [w810 TRUE] -> w796
                  tunnel: w794 -> [w809 _]
                  frame False {
                    n340 = Not Equal?(x=w809, y=w815) -> (x != y?=w813:bool)
                    n341 = Select(t=TRUE, s=w813, f=FALSE) -> (s? t:f=w810:bool)
                  }
                  frame True {
                  }
                }
                n342 = Compound Arithmetic op=OR(w800, TRUE ("value")) -> (w799:bool)
                n343 = Build Array(w798, w795) -> (w797:i32[])
              }
              n344 = while {
                tunnel: w664 -> [w856]
                shift-right: [w848] -> _
                shift-left: w662 -> [w857]
                shift-right: [w845] -> _
                shift-left: w663 -> [w858]
                tunnel: [w847] -> w668 mode=indexing if=w846
                tunnel: w661 -> [w844]
                stop <- w849 stop-if-true
                n345 = Increment(x=w857) -> (x+1=w848:i32)
                n346 = Increment(x=w858) -> (x+1=w845:i32)
                n347 = Index Array(array=w856, index (row)=w848, index (col)=w845) -> (element=w855:T1)
                n348 = Unbundle By Name(w855) -> ("Piece.Color"=w851:T2, "Piece.Type"=w854:T4)
                n349 = Equal?(x=#typedef_PieceType."None", y=w854) -> (x = y?=w852:bool)
                n350 = case shown="False" w852 {
                  tunnel: w851 -> [w865 _]
                  tunnel: [TRUE FALSE] -> w850
                  tunnel: [w860 TRUE] -> w846
                  tunnel: w844 -> [w859 _]
                  frame False {
                    n351 = Not Equal?(x=w859, y=w865) -> (x != y?=w863:bool)
                    n352 = Select(t=TRUE, s=w863, f=FALSE) -> (s? t:f=w860:bool)
                  }
                  frame True {
                  }
                }
                n353 = Compound Arithmetic op=OR(w850, TRUE ("value")) -> (w849:bool)
                n354 = Build Array(w848, w845) -> (w847:i32[])
              }
              n355 = while {
                tunnel: w664 -> [w831]
                shift-right: [w823] -> _
                shift-left: w662 -> [w832]
                shift-right: [w820] -> _
                shift-left: w663 -> [w833]
                tunnel: [w822] -> w667 mode=indexing if=w821
                tunnel: w661 -> [w819]
                stop <- w824 stop-if-true
                n356 = Increment(x=w832) -> (x+1=w823:i32)
                n357 = Decrement(x=w833) -> (x-1=w820:i32)
                n358 = Index Array(array=w831, index (row)=w823, index (col)=w820) -> (element=w830:T1)
                n359 = Unbundle By Name(w830) -> ("Piece.Color"=w826:T2, "Piece.Type"=w829:T4)
                n360 = Equal?(x=#typedef_PieceType."None", y=w829) -> (x = y?=w827:bool)
                n361 = case shown="False" w827 {
                  tunnel: w826 -> [w840 _]
                  tunnel: [TRUE FALSE] -> w825
                  tunnel: [w835 TRUE] -> w821
                  tunnel: w819 -> [w834 _]
                  frame False {
                    n362 = Not Equal?(x=w834, y=w840) -> (x != y?=w838:bool)
                    n363 = Select(t=TRUE, s=w838, f=FALSE) -> (s? t:f=w835:bool)
                  }
                  frame True {
                  }
                }
                n364 = Compound Arithmetic op=OR(w825, TRUE ("value")) -> (w824:bool)
                n365 = Build Array(w823, w820) -> (w822:i32[])
              }
              n366 = Insert Into Array(array=w668, new element #1=w667, new element #2=w666, new element #3=w665, new element #4=w660, new element #5=w659, new element #6=w658, new element #7=w657) -> (w656:i32[][])  [unwired: 2 in]
            }
          }
        }
      }
      n367 = Equal?(x=w16, y=i32[][] [[-1]] ("x")) -> (x = y?=w19:bool[][])
      n368 = Or Array Elements(Boolean array=w19) -> (logical OR=w18:bool)
      n369 = case shown="False" w18 {
        tunnel: w17 -> [w31 w34]
        tunnel: w16 -> [_ w33]
        tunnel: [w31 w32] -> w15
        frame True {
        }
        frame False {
          n370 = for {
            tunnel: w33 -> [w41] mode=indexing
            shift-right: [w35] -> w32
            shift-left: w34 -> [w42]
            n371 = Index Array(array=w41, index #1=0 ("index"), index #2=1 ("index")) -> (element #1=w38:i32, element #2=w37:i32)
            n372 = Replace Array Subset(array=w42, new element=TRUE ("new element/subarray"), index (row)=w38, index (col)=w37) -> (w35:bool[][])
          }
        }
      }
    }
  }
  "Attacked Squares" <- w7
